vi "Error Channels Write.vi"   [LabVIEW 2023, in "Chiller.lvclass"]
uses:
  Chiller.lvclass
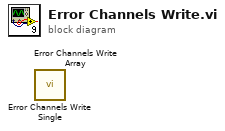
[diagram p0: block diagram]
diagram:
  n1 = call "Error Channels Write Single.vi"() -> ()  [unwired: 10 in, 2 out]
  n2 = call "Error Channels Write Array.vi"() -> ()  [unwired: 10 in, 2 out]
